vi "Set_SJ_Amplitude.vi"() -> (5 "Plug in titles":string[](array[string])=["Synthetic_Jet:Frequency:Hz", "Syntehtic_Jet:Amplitude:V", "Synthetic_Jet:Target:Value"], 7 "Plug in values":string[](array[string])=["0.032033", "-0.000033"])   [LabVIEW 2022 SP3]
uses:
  Globals/Meas_global.vi
  Globals/Synthetic_jet_global.vi
  <vilib>/measure/matone.llb/Extract Single Tone Information 1 Chan.vi
  <vilib>/measure/NI_MAPro.lvlib
panel:
  out "Error":dbl=-3.314787923475865e-05
  out "Error":cluster{"Frequency Array":dbl[], dbl[]}(graph)={"Frequency Array"=[300.0, 333.3333333333333, 366.6666666666667, 400.0, 433.3333333333333, 466.6666666666667, 500.0, 533.3333333333334, 566.6666666666666, 600.0, 633.3333333333334, 666.6666666666666, 700.0, 733.3333333333334, 766.6666666666666, 800.0, 833.3333333333334, 866.6666666666666, 900.0, 933.3333333333334, 966.6666666666666, 1000.0, 1033.3333333333333, 1066.6666666666667, 1100.0], [0.0016499991392928612, 0.001194305674718489, 0.0005038967799521829, 0.0004168601031609154, -4.707633877185785e-05, -2.5779934509626012e-05, -2.25266718581682e-05, -3.594337655055124e-05, -2.8642908492554353e-05, -3.292714538750269e-05, -4.608438710474588e-05, -3.911815513831657e-05, 3.764978775293304e-06, -2.8057984966876892e-05, 4.21391640583052e-05, 1.7037183298533598e-05, 1.954309115251296e-05, -4.14668782148242e-05, -4.7804719161451126e-05, -2.5595818681320437e-05, -4.697149168106374e-05, -1.7553576966894413e-05, -4.4593927105915365e-05, -1.534886743465025e-05, -3.314787923475865e-05]}
  out "Amplitude":cluster{dbl[], dbl[]}(graph)
  out "Attempted New Amplitude":dbl=71.78690646050504
  out "Function generator Amplitude":dbl=0.9837455447108608
  out "Current Amplitude":dbl=71.81342476389284
  out "Max Displacement":dbl=0.03203314787923476
  out "Displacement":cluster{"Frequency Array":dbl[], dbl[]}[](graph)=[{"Frequency Array"=array[219 elements], array[219 elements]}, {"Frequency Array"=[300.0, 333.3333333333333, 366.6666666666667, 400.0, 433.3333333333333, 466.6666666666667, 500.0, 533.3333333333334, 566.6666666666666, 600.0, 633.3333333333334, 666.6666666666666, 700.0, 733.3333333333334, 766.6666666666666, 800.0, 833.3333333333334, 866.6666666666666, 900.0, 933.3333333333334, 966.6666666666666, 1000.0, 1033.3333333333333, 1066.6666666666667, 1100.0], [0.03035000086070714, 0.03080569432528151, 0.03149610322004782, 0.031583139896839085, 0.03204707633877186, 0.03202577993450963, 0.03202252667185817, 0.03203594337655055, 0.032028642908492555, 0.0320329271453875, 0.03204608438710475, 0.03203911815513832, 0.03199623502122471, 0.03202805798496688, 0.031957860835941695, 0.03198296281670147, 0.03198045690884749, 0.032041466878214825, 0.03204780471916145, 0.03202559581868132, 0.032046971491681064, 0.032017553576966895, 0.032044593927105916, 0.03201534886743465, 0.03203314787923476]}]
  in  "VISA resource name":refnum<visa-resource-name>="USB0::0x0699::0x0347::C036837::INSTR"
  out "New Amplitude":dbl=71.78690646050504
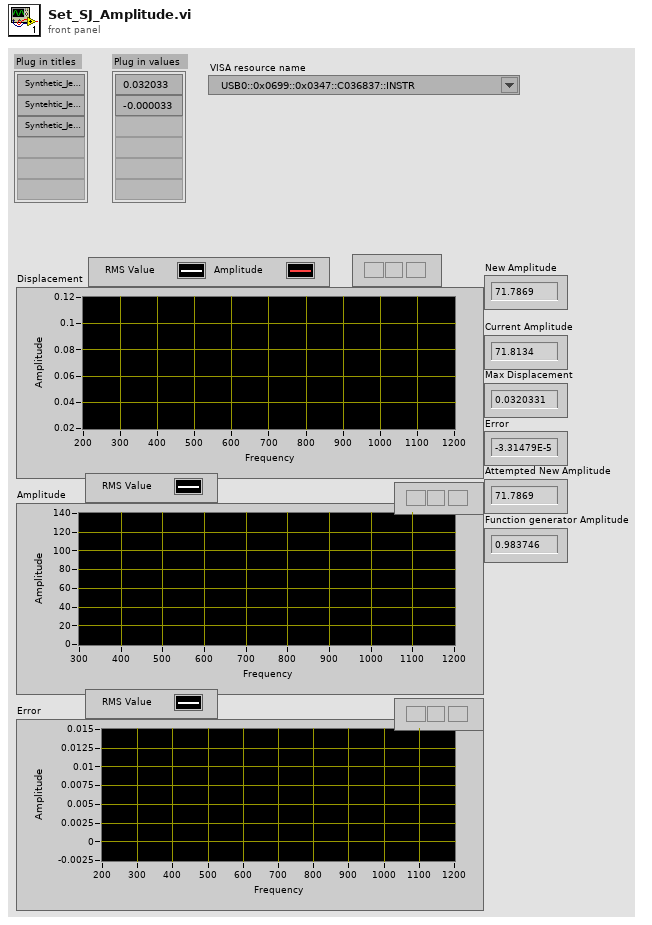
[diagram p1: front panel]
types:
  T1 = typedef "Analysis_info_cluster.ctl" = cluster{"Colour":u32, "Inst type":T2, "Inst name":string, "Symbol":string, "Code name":string, "Extra Info":string, "Inst Array":T3, "Extra Titles":string[], "Extra Values":string[], "U":dbl, "u^2":dbl, "u^3":dbl, "u^4":dbl, "Skew_u":dbl, "Kurt_u":dbl, "Sd Error in Mean":dbl, "% u'/U":dbl, "X":dbl, "Y":dbl, "Z":dbl, "Timescale integral Estimate":dbl, "Sd Error in Variance":dbl, "Calib File":path, "Calib Constants":dbl[], "Output Position":bool, "Stats":enum16{"None", "Basic", "Full"}, "Av Sampling Rate":dbl, "Av No of Samples":dbl, "Total Meas Time (s)":dbl, "ADAM Ch Name":string, "Max value":dbl, "Min value":dbl, "Req Sample Rate Hz":dbl, "Sync Delay Time (s)":dbl, "Ch No":i16, "Device":string, "Use Latest Calib":bool, "Port":string, "Metadata Ch Names":string[], "Metadata Ch Values":string[], "Label":string}
  T2 = typedef "Inst_type.ctl" = enum16{"Raw voltage", "Raw with zero offsetting", "Propeller anemometer", "Pressure Transducer", "Pitot-static tube", "Hot wire", "Cross wire 1", "Cross wire 2", "Generic Linear", "Generic Polynomial", "Generic BackPoly", "Fast FID", "Thermocouple", "Cold wire", "Pulsed Wire", "LDA Vel", "LDA Tran time", "LDA Arr time", "Microphone"}
  T3 = typedef "Instrument_Array.ctl" = enum16{"PWA", "LDA", "Analogue"}
  T4 = typedef "Post_Process.ctl" = enum16{"Take New Data", "Post Process Raw Data File"}
  T5 = typedef "Time_Trace_Cluster.ctl" = cluster{"Weighting":dbl[], "Voltage":dbl[], "Eng Values":dbl[]}
  T6 = enum32{"none", "input signal", "detected signal", "residual signal"}
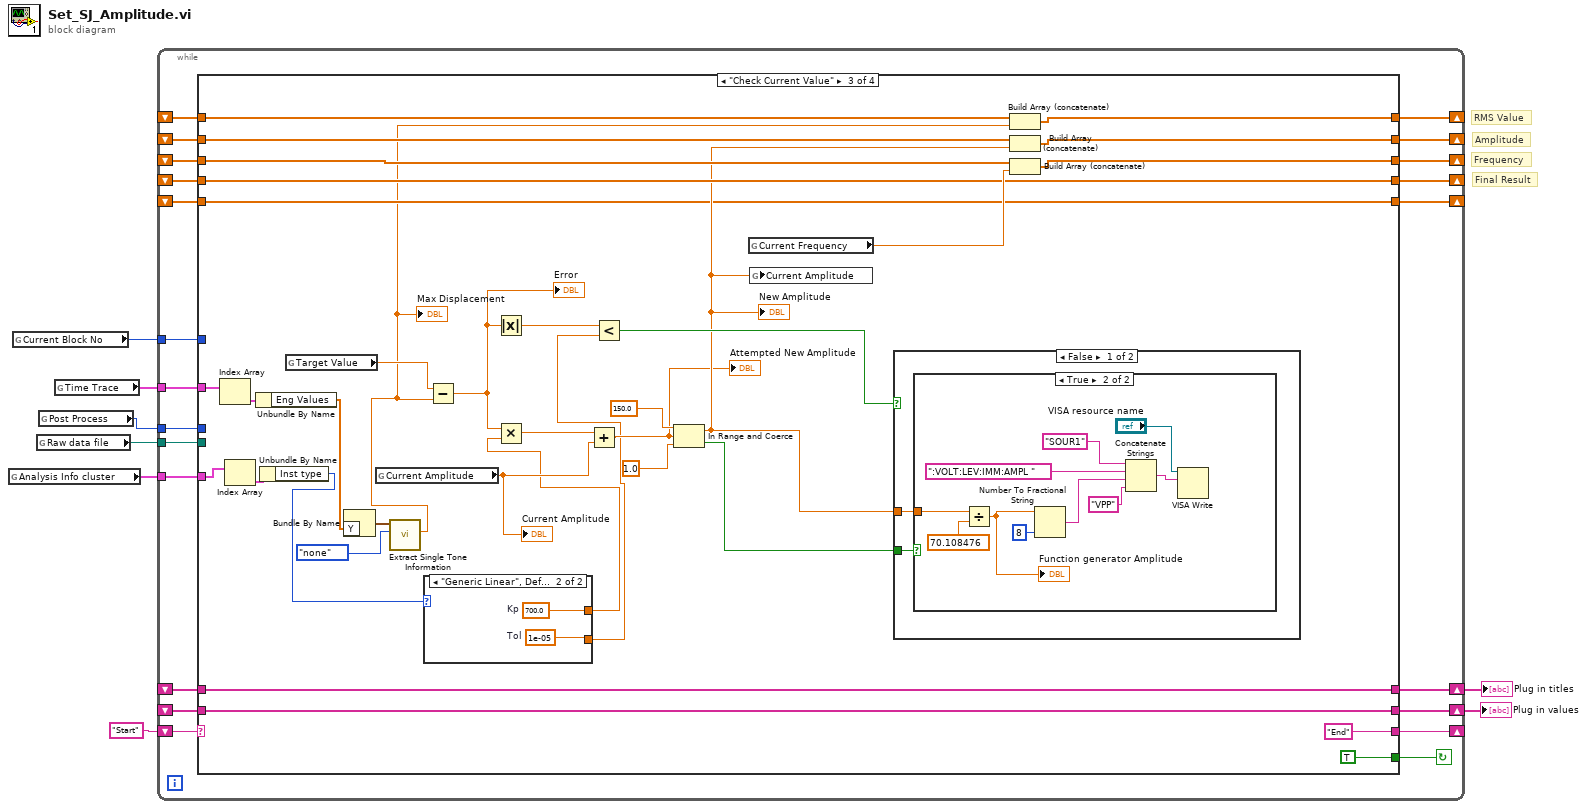
[diagram p0: block diagram]
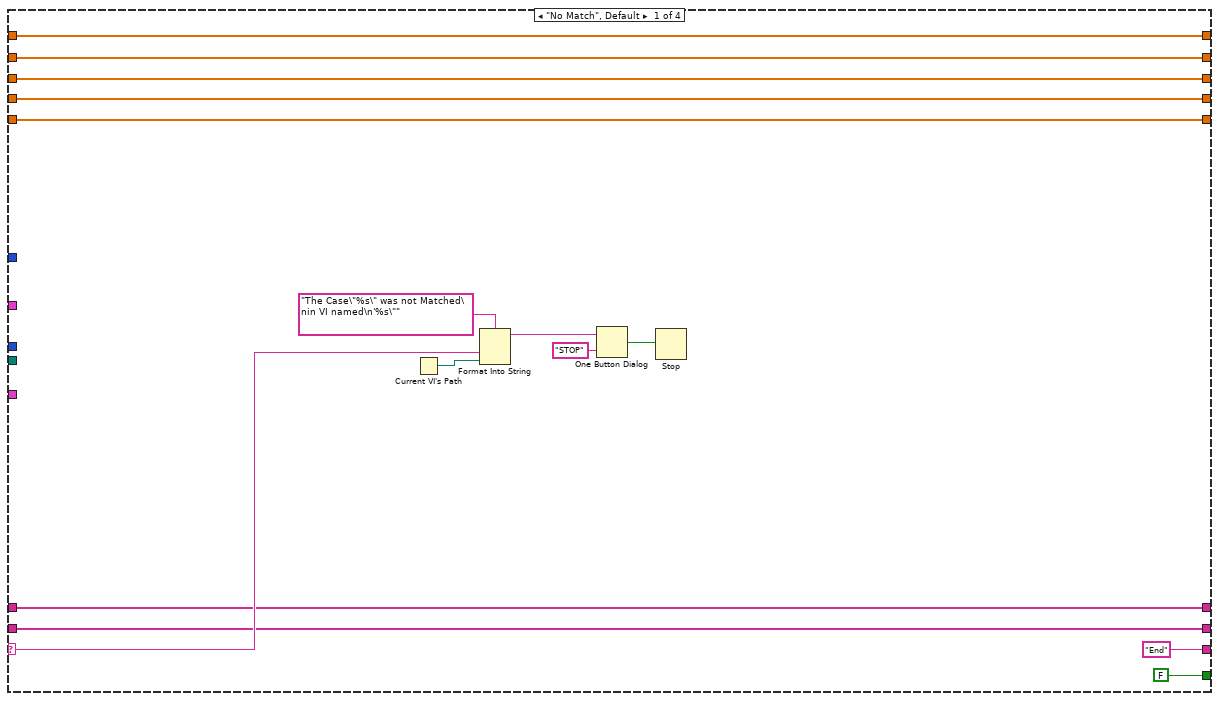
[diagram p2: hidden frame]
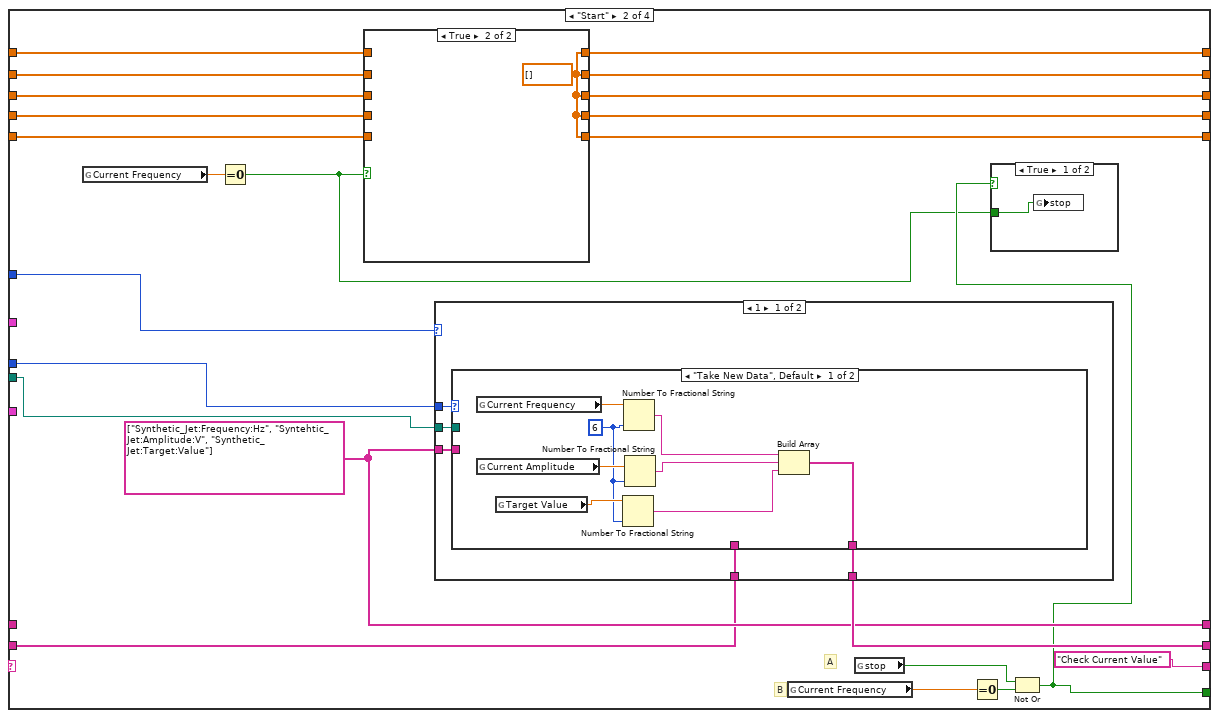
[diagram p3: hidden frame]
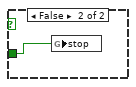
[diagram p4: hidden frame]
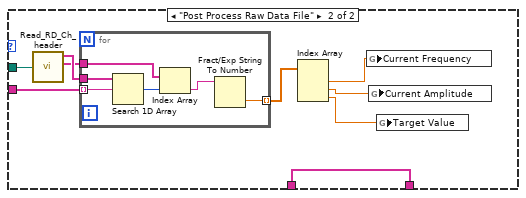
[diagram p6: hidden frame]
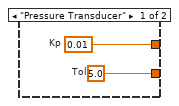
[diagram p8: hidden frame]
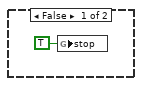
[diagram p9: hidden frame]
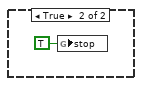
[diagram p10: hidden frame]
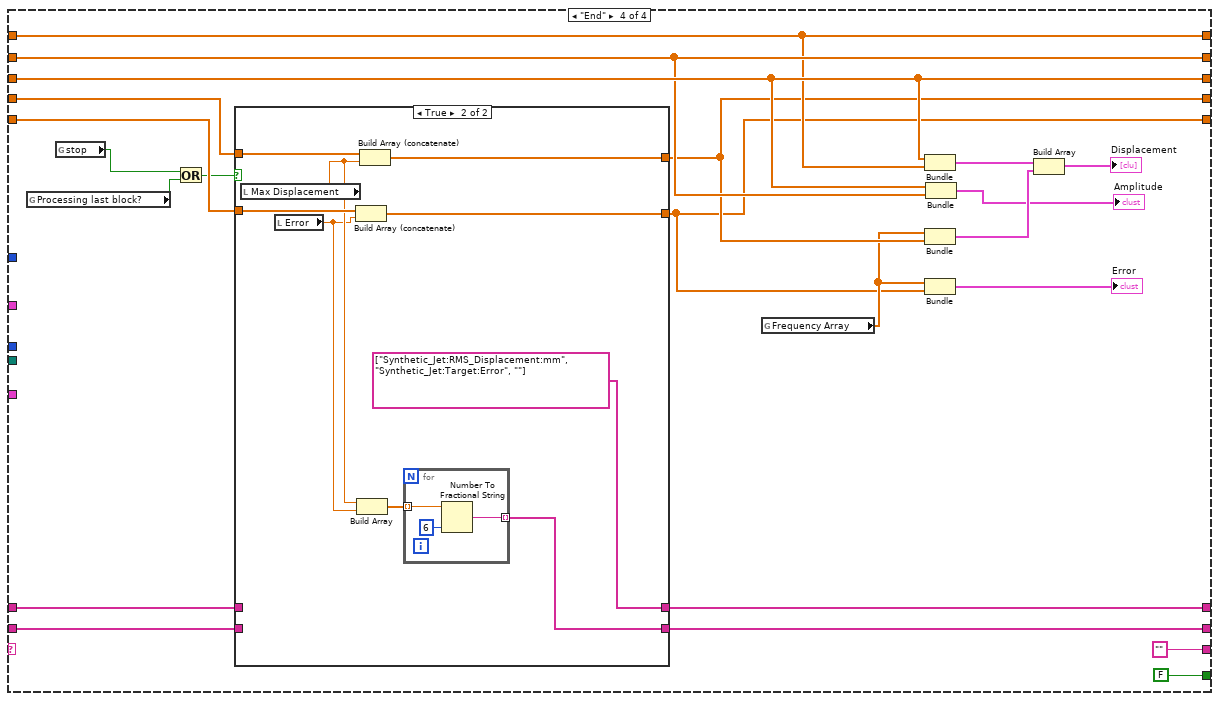
[diagram p11: hidden frame]
diagram:
  # "Final Result"
  # "Frequency"
  # "Amplitude"
  # "RMS Value"
  n1 = global read "Meas_global.vi" "Analysis Info cluster"() -> (w1:T1[])
  n2 = global read "Meas_global.vi" "Current Block No"() -> (w7:i32)
  n3 = global read "Meas_global.vi" "Raw data file"() -> (w4:path)
  n4 = global read "Meas_global.vi" "Post Process"() -> (w5:T4)
  n5 = global read "Meas_global.vi" "Time Trace"() -> (w6:T5[])
  n6 = while {
    shift-right: [w28] -> _
    shift-left: "Start" -> [w29]
    tunnel: w7 -> [w27]
    tunnel: w6 -> [w26]
    tunnel: w5 -> [w25]
    tunnel: w4 -> [w24]
    shift-right: [w22] -> w3
    shift-left: _ -> [w23]
    shift-right: [w21] -> w2
    shift-left: _ -> [w20]
    shift-right: [w19] -> _
    shift-left: _ -> [w18]
    shift-right: [w17] -> _
    shift-left: _ -> [w16]
    shift-right: [w15] -> _
    shift-left: _ -> [w14]
    shift-right: [w13] -> _
    shift-left: _ -> [w12]
    shift-right: [w10] -> _
    shift-left: _ -> [w11]
    tunnel: w1 -> [w9]
    stop <- w30 continue-if-true
    n7 = case shown="\"Check Current Value\"" w29 {
      selector: w29 -> [w40 _ _ _]
      tunnel: [FALSE w49 TRUE FALSE] -> w30
      tunnel: ["End" "Check Current Value" "End" ""] -> w28
      tunnel: w27 -> [_ w62 _ _]
      tunnel: w26 -> [_ _ w136 _]
      tunnel: w25 -> [_ w67 _ _]
      tunnel: w24 -> [_ w63 _ _]
      tunnel: [w37 w65 w138 w160] -> w22
      tunnel: w23 -> [w37 _ w138 w162]
      tunnel: [w36 w66 w137 w159] -> w21
      tunnel: w20 -> [w36 w64 w137 w161]
      tunnel: [w35 w57 w129 w173] -> w19
      tunnel: w18 -> [w35 w56 w131 w173]
      tunnel: [w34 w59 w132 w172] -> w17
      tunnel: w16 -> [w34 w58 w130 w172]
      tunnel: [w33 w55 w128 w175] -> w15
      tunnel: w14 -> [w33 w54 w127 w175]
      tunnel: [w32 w52 w125 w171] -> w13
      tunnel: w12 -> [w32 w51 w125 w176]
      tunnel: w11 -> [w31 w46 w121 w169]
      tunnel: [w31 w47 w121 w166] -> w10
      tunnel: w9 -> [_ _ w110 _]
      frame "No Match", Default {
        n8 = Current VI's Path() -> (path=w45:path)
        n9 = Format Into String(format string="The Case\"%s\" was not Matched\nin VI named\n'%s\"" ("Format String"), w40, w45) -> (resulting string=w42:string)  [unwired: 2 in, 1 out]
        n10 = One Button Dialog(message=w42, button name ("OK")="STOP") -> (true=w44:bool)
        n11 = Stop(stop? (T)=w44) -> ()
      }
      frame "Start" {
        w65 = string[] ["Synthetic_Jet:Frequency:Hz", "Syntehtic_Jet:Amplitude:V", "Synthetic_Jet:Target:Value"] ("Desired Ch Names")
        # "B"
        # "A"
        n12 = global read "Synthetic_jet_global.vi" "Current Frequency"() -> (w60:dbl)
        n13 = Equal To 0?(x=w60) -> (x = 0?=w48:bool)
        n14 = case shown="True" w48 {
          tunnel: [w75 w76] -> w59
          tunnel: w58 -> [w75 _]
          tunnel: [w74 w76] -> w57
          tunnel: w56 -> [w74 _]
          tunnel: [w73 w76] -> w55
          tunnel: w54 -> [w73 _]
          tunnel: [w72 w76] -> w52
          tunnel: w51 -> [w72 _]
          tunnel: [w71 w76] -> w47
          tunnel: w46 -> [w71 _]
          frame False {
          }
          frame True {
            w76 = dbl[] []
          }
        }
        n15 = case shown="1" w62 {
          tunnel: w67 -> [w81 _]
          tunnel: [w80 w105] -> w66
          tunnel: w65 -> [w79 _]
          tunnel: w64 -> [w78 w105]
          tunnel: w63 -> [w77 _]
          frame 1 {
            n16 = case shown="\"Take New Data\", Default" w81 {
              tunnel: w79 -> [_ w96]
              tunnel: [w87 w95] -> w80
              tunnel: w78 -> [_ w95]
              tunnel: w77 -> [_ w94]
              frame "Take New Data", Default {
                w83 = i16 6 ("precision (6)")
                n17 = global read "Synthetic_jet_global.vi" "Current Frequency"() -> (w89:dbl)
                n18 = global read "Synthetic_jet_global.vi" "Current Amplitude"() -> (w86:dbl)
                n19 = global read "Synthetic_jet_global.vi" "Target Value"() -> (w84:dbl)
                n20 = Number To Fractional String(number=w84, precision (6)=w83) -> (F-format string=w82:string)  [unwired: 2 in]
                n21 = Number To Fractional String(number=w89, precision (6)=w83) -> (F-format string=w88:string)  [unwired: 2 in]
                n22 = Number To Fractional String(number=w86, precision (6)=w83) -> (F-format string=w85:string)  [unwired: 2 in]
                n23 = Build Array(w88, w85, w82) -> (w87:string[])
              }
              frame "Post Process Raw Data File" {
                n24 = call "Read_RD_Ch_header.vi"("Raw data file"=w94) -> ("Ch Name Out"=w98:string[], "Ch Values"=w97:string[])  [unwired: 2 out]
                n25 = for {
                  tunnel: w98 -> [w104]
                  tunnel: w97 -> [w103]
                  tunnel: w96 -> [w101] mode=indexing
                  tunnel: [w99] -> w93 mode=indexing
                  n26 = Search 1D Array(1D array=w104, element=w101) -> (index of element=w102:i32)  [unwired: 1 in]
                  n27 = Index Array(array=w103, index=w102) -> (element=w100:string)
                  n28 = Fract/Exp String To Number(string=w100) -> (number=w99:dbl)  [unwired: 3 in, 1 out]
                }
                n29 = Index Array(array=w93) -> (element #1=w92:dbl, element #2=w90:dbl, element #3=w91:dbl)  [unwired: 3 in]
                n30 = global write "Synthetic_jet_global.vi" "Current Frequency"(w92) -> ()
                n31 = global write "Synthetic_jet_global.vi" "Current Amplitude"(w90) -> ()
                n32 = global write "Synthetic_jet_global.vi" "Target Value"(w91) -> ()
              }
            }
          }
          frame 2, Default {
          }
        }
        n33 = global read "Synthetic_jet_global.vi" "Current Frequency"() -> (w61:dbl)
        n34 = global read "Meas_global.vi" "stop"() -> (w50:bool)
        n35 = Equal To 0?(x=w61) -> (x = 0?=w53:bool)
        n36 = Not Or(1:w53, 2:w50) -> (0:w49:bool)
        n37 = case shown="True" w49 {
          tunnel: w48 -> [w69 w70]
          frame True {
            n38 = global write "Meas_global.vi" "stop"(w69) -> ()
          }
          frame False {
            n39 = global write "Meas_global.vi" "stop"(w70) -> ()
          }
        }
      }
      frame "Check Current Value" {
        n40 = Index Array(array=w136) -> (element=w135:T5)  [unwired: 1 in]
        n41 = Index Array(array=w110) -> (element=w109:T1)  [unwired: 1 in]
        n42 = Unbundle By Name(w135) -> ("Eng Values"=w114:dbl[])
        n43 = Unbundle By Name(w109) -> ("Inst type"=w108:T2)
        n44 = global read "Synthetic_jet_global.vi" "Target Value"() -> (w117:dbl)
        n45 = Bundle By Name("Y"=w114) -> (w113:waveform(dbl))  [unwired: 1 in]
        n46 = global read "Synthetic_jet_global.vi" "Current Amplitude"() -> (w118:dbl)
        "Current Amplitude" <- w118
        n47 = call-poly <vilib>:"Extract Single Tone Information.vi"("export mode"=T6."none", "time signal in"=w113) -> ("detected amplitude"=w111:dbl)  [unwired: 4 in, 5 out]
        "Max Displacement" <- w111
        n48 = case shown="\"Generic Linear\", Default" w108 {
          tunnel: [w142 w144] -> w107
          tunnel: [w141 w143] -> w106
          frame "Pressure Transducer" {
            w141 = 5.0  # Tol
            w142 = 0.01  # Kp
          }
          frame "Generic Linear", Default {
            w143 = 1e-05  # Tol
            w144 = 700.0  # Kp
          }
        }
        n49 = Subtract(x=w117, y=w111) -> (x-y=w116:dbl)
        "Error" <- w116
        n50 = Absolute Value(x=w116) -> (abs(x)=w115:dbl)
        n51 = Multiply(x=w116, y=w107) -> (x*y=w119:dbl)
        n52 = Add(x=w119, y=w118) -> (x+y=w120:dbl)
        "Attempted New Amplitude" <- w120
        n53 = Less?(x=w115, y=w106) -> (x < y?=w124:bool)
        n54 = In Range and Coerce(upper limit=150.0, x=w120, lower limit=1.0) -> (coerced(x)=w122:dbl, In Range?=w123:bool)
        "New Amplitude" <- w122
        n55 = global read "Synthetic_jet_global.vi" "Current Frequency"() -> (w126:dbl)
        n56 = global write "Synthetic_jet_global.vi" "Current Amplitude"(w122) -> ()
        n57 = case shown="False" w124 {
          tunnel: w122 -> [w146 _]
          tunnel: w123 -> [w145 _]
          frame False {
            n58 = case shown="True" w145 {
              tunnel: w146 -> [_ w150]
              frame False {
                n59 = global write "Meas_global.vi" "stop"(TRUE ("stop")) -> ()
              }
              frame True {
                n60 = Divide(x=w150, y=70.108476) -> (x/y=w148:dbl)
                "Function generator Amplitude" <- w148
                n61 = Number To Fractional String(number=w148, precision (6)=i16 8) -> (F-format string=w153:string)  [unwired: 2 in]
                n62 = Concatenate Strings("SOUR1" ("string"), ":VOLT:LEV:IMM:AMPL " ("string"), w153, "VPP" ("string")) -> (w154:string)
                n63 = VISA Write(VISA resource name="VISA resource name", write buffer=w154) -> ()  [unwired: 1 in, 3 out]
              }
            }
          }
          frame True {
            n64 = global write "Meas_global.vi" "stop"(TRUE ("stop")) -> ()
          }
        }
        n65 = Build Array (concatenate)(w130, w111) -> (w132:dbl[])
        n66 = Build Array (concatenate)(w131, w122) -> (w129:dbl[])
        n67 = Build Array (concatenate)(w127, w126) -> (w128:dbl[])
      }
      frame "End" {
        n68 = global read "Meas_global.vi" "Processing last block?"() -> (w164:bool)
        n69 = global read "Meas_global.vi" "stop"() -> (w165:bool)
        n70 = Or(x=w165, y=w164) -> (x .or. y?=w163:bool)
        n71 = case shown="True" w163 {
          tunnel: w176 -> [w184 w193]
          tunnel: [w184 w192] -> w171
          tunnel: w169 -> [w183 w191]
          tunnel: [w183 w190] -> w166
          tunnel: w162 -> [w182 _]
          tunnel: w161 -> [w181 _]
          tunnel: [w182 string[] ["Synthetic_Jet:RMS_Displacement:mm", "Synthetic_Jet:Target:Error", ""] ("Desired Ch Names")] -> w160
          tunnel: [w181 w185] -> w159
          frame False {
          }
          frame True {
            n72 = local read "Max Displacement"() -> (w187:dbl)
            n73 = local read "Error"() -> (w186:dbl)
            n74 = Build Array (concatenate)(w191, w186) -> (w190:dbl[])
            n75 = Build Array(w187, w186) -> (w188:dbl[])
            n76 = Build Array (concatenate)(w193, w187) -> (w192:dbl[])
            n77 = for {
              tunnel: w188 -> [w195] mode=indexing
              tunnel: [w194] -> w185 mode=indexing
              n78 = Number To Fractional String(number=w195, precision (6)=i16 6) -> (F-format string=w194:string)  [unwired: 2 in]
            }
          }
        }
        n79 = global read "Synthetic_jet_global.vi" "Frequency Array"() -> (w168:dbl[])
        n80 = Bundle(w175, w172) -> (w178:cluster{dbl[], dbl[]})  [unwired: 1 in]
        n81 = Bundle("Frequency Array"=w168, w171) -> (w174:cluster{"Frequency Array":dbl[], dbl[]})  [unwired: 1 in]
        n82 = Bundle("Frequency Array"=w168, w166) -> (→"Error":cluster{"Frequency Array":dbl[], dbl[]})  [unwired: 1 in]
        n83 = Bundle(w175, w173) -> (→"Amplitude":cluster{dbl[], dbl[]})  [unwired: 1 in]
        n84 = Build Array(w178, w174) -> (→"Displacement":cluster{"Frequency Array":dbl[], dbl[]}[])
      }
    }
  }
  "Plug in values" <- w2
  "Plug in titles" <- w3
